vi "公式复合写入.vi"(8 "公式":cluster{"X^2":dbl, "X":dbl, "b":dbl}, 9 "量程下拉列表":enum16{"低量程", "高量程"}(ring), 10 "测量模式":enum16{"跨度核查", "水样测量", "零点核查", "标样核查", "加标回收"}(ring), 11 "参数下拉列表":u16(ring)) -> ()   [LabVIEW 2016, in "斯坦道氨氮V2.lvlib"]
uses:
  <vilib>/Utility/miscctls.llb/LVPointTypeDef.ctl
panel:
  in  "读取":bool
  in  "一键写入":bool=TRUE
  out "连接的字符串":string
  in  "关闭":bool
  in  "写入":bool
  # "请选择要写入的参数"
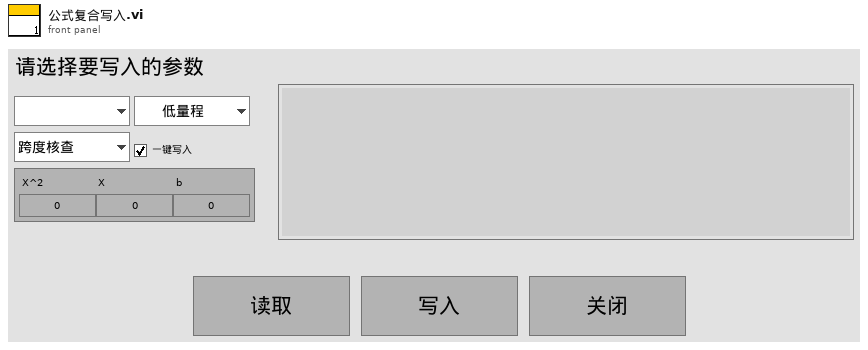
[diagram p1: front panel]
types:
  T1 = typedef "LVPointTypeDef.ctl" = cluster{"Horizontal":i16, "Vertical":i16}
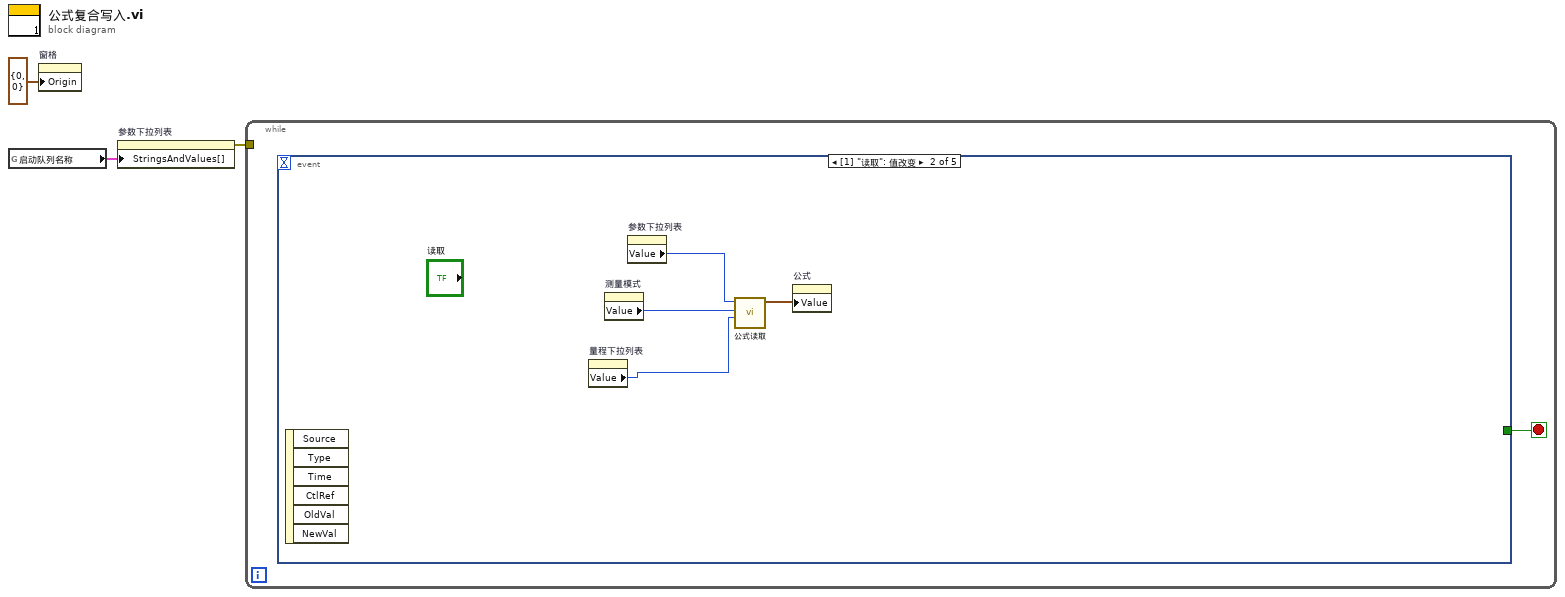
[diagram p0: block diagram]
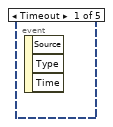
[diagram p2: hidden frame]
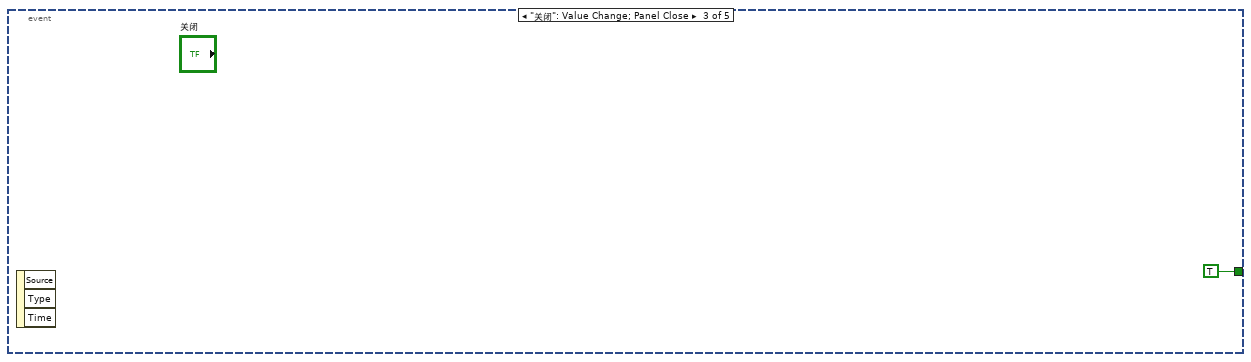
[diagram p3: hidden frame]
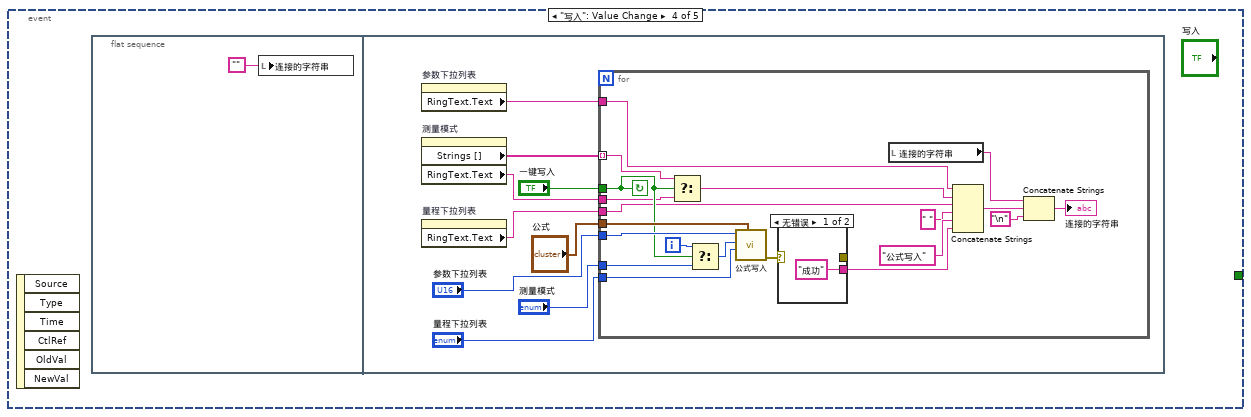
[diagram p4: hidden frame]
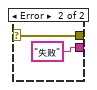
[diagram p5: hidden frame]
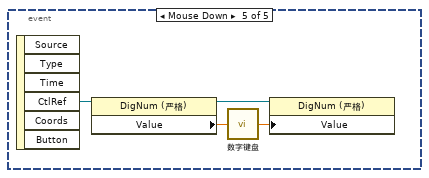
[diagram p6: hidden frame]
diagram:
  n1 = global read "总磷总氮断电保存全局变量.vi" "启动队列名称"() -> (w2:cluster{"String":string, "Value":u16}[])
  n2 = property on="窗格" class="Pane"("Origin"=T1 {"Horizontal"=0, "Vertical"=0} ("原点")) -> ()  [unwired: 2 in, 2 out]
  n3 = property on="参数下拉列表" class="Ring (严格)"("StringsAndValues[]"=w2) -> (error out=w1:errorcluster)  [unwired: 2 in, 1 out]
  n4 = while {
    tunnel: w1 -> [_]
    stop <- w4 stop-if-true
    n5 = event shown="[1] \"读取\": 值改变" {
      selector: _ -> [_ _ _ _ _]
      dyn-events: _ -> [_ _ _ _ _]
      timeout: _ -> [_ _ _ _ _]
      tunnel: [_ _ TRUE _ _] -> w4
      event Timeout {
        n6 = event-data() -> ()  [unwired: 1 in, 3 out]
      }
      event "读取": Value Change {
        n7 = event-data() -> ()  [unwired: 1 in, 6 out]
        n8 = property on="量程下拉列表" class="Enum (严格)"() -> ("Value"=w6:enum16{"低量程", "高量程"})  [unwired: 2 in, 2 out]
        n9 = property on="测量模式" class="Enum (严格)"() -> ("Value"=w7:enum16{"跨度核查", "水样测量", "零点核查", "标样核查", "加标回收"})  [unwired: 2 in, 2 out]
        n10 = property on="参数下拉列表" class="Ring (严格)"() -> ("Value"=w8:u16)  [unwired: 2 in, 2 out]
        n11 = call "公式读取.vi"("量程下拉列表"=w6, "测量模式"=w7, "参数下拉列表"=w8) -> ("公式"=w5:cluster{"X^2":dbl, "X":dbl, "b":dbl})  [unwired: 7 in, 1 out]
        n12 = property on="公式" class="Clust (严格)"("Value"=w5) -> ()  [unwired: 2 in, 2 out]
      }
      event "关闭": Value Change; Panel Close {
        n13 = event-data() -> ()  [unwired: 1 in, 3 out]
      }
      event "写入": Value Change {
        n14 = event-data() -> ()  [unwired: 1 in, 6 out]
        n15 = flat-sequence {
          frame #0 {
            n16 = local write "连接的字符串"("") -> ()
          }
          frame #1 {
            n17 = property on="参数下拉列表" class="Ring (严格)"() -> ("RingText.Text"=w12:string)  [unwired: 2 in, 2 out]
            n18 = property on="测量模式" class="Enum (严格)"() -> ("Strings []"=w16:string[], "RingText.Text"=w15:string)  [unwired: 2 in, 2 out]
            n19 = property on="量程下拉列表" class="Enum (严格)"() -> ("RingText.Text"=w11:string)  [unwired: 2 in, 2 out]
            n20 = for {
              tunnel: "公式" -> [w39]
              tunnel: "参数下拉列表" -> [w35]
              tunnel: "量程下拉列表" -> [w38]
              tunnel: w16 -> [w31] mode=indexing
              tunnel: w15 -> [w30]
              tunnel: "一键写入" -> [w32]
              tunnel: "测量模式" -> [w34]
              tunnel: w12 -> [w22]
              tunnel: w11 -> [w20]
              i -> [w36]
              stop <- w32 continue-if-true
              n21 = Select(t=w31, s=w32, f=w30) -> (s? t:f=w24:string)
              n22 = Select(t=w36, s=w32, f=w34) -> (s? t:f=w33:i32)
              n23 = call "公式写入.vi"("公式"=w39, "量程下拉列表"=w38, "测量模式"=w33, "参数下拉列表"=w35) -> ("error out"=w37:errorcluster)  [unwired: 7 in]
              n24 = case shown="无错误" w37 {
                selector: w37 -> [_ w42]
                tunnel: [_ w42] -> _
                tunnel: ["成功" "失败"] -> w23
                frame No Error {
                }
                frame Error {
                }
              }
              n25 = local read "连接的字符串"() -> (w25:string)
              n26 = Concatenate Strings(w22, w24, w20, " " ("字符串"), "公式写入", w23) -> (w28:string)
              n27 = Concatenate Strings(w25, w28, "\n") -> (→"连接的字符串":string)
            }
          }
        }
      }
      event "公式.X^2", "公式.X", "公式.b": Mouse Down {
        n28 = event-data() -> ("CtlRef"=w46:refnum<vi>)  [unwired: 1 in, 5 out]
        n29 = property class="DigNum (严格)"(reference=w46) -> (reference out=w43:refnum<vi>, "Value"=w45:dbl)  [unwired: 1 in, 1 out]
        n30 = call "数字键盘.vi"("OldNumber"=w45) -> ("NewNumber"=w44:dbl)
        n31 = property class="DigNum (严格)"(reference=w43, "Value"=w44) -> ()  [unwired: 1 in, 2 out]
      }
    }
  }
